vi "CRYAna Harmonic.vi"(0 "Calibration Response Cluster":T1={"Calibration"={"Calibration Step Name"="", "Device"="", "Correction Curve Name"="", "Equalization Curve Name"="", "Sensitivity Curve Name"="", "Corr Folder and File"="", "EQ Folder and File"="", "Sens Folder and File"="", "Corr Step size"=0, "EQ Step size"=0, "Input"=FALSE, "Last Cal Date (sec)"=timestamp(0 s since 1904-01-01), "Cha Name"="", "Corr Curve Found"=FALSE, "EQ Curve Found"=FALSE, "Sens Curve Found"=FALSE, "Signal Type"="", "Calibrated Device"="", "Hz"=0}, "Corr Curve"={"Name"="", "Curve"=[], "X data"=1, "Y data"=1, "Z data"=1, "X axis"=0, "Y axis"=1, "Z axis"=1, "X unit"="Hz", "Y unit"="", "Z unit"="deg.", "X dB ref"=1.0, "Y dB ref"=1.0, "Z dB ref"=1.0, "single val"=FALSE, "protected"=FALSE, "display X"=TRUE, "display Y"=TRUE, "display Z"=TRUE, "Test Info"="", "Step No."=0, "Plot Settings"={"Color"=0, "Interpolation"=0, "Point Style"=0, "Line Style"=0, "Point Color"=0, "Line Width"=0, "Bar Plot Style"=0, "Fill To"=0}, "AutoProtect"=FALSE}, "EQ Curve"={"Name"="", "Curve"=[], "X data"=1, "Y data"=1, "Z data"=1, "X axis"=0, "Y axis"=1, "Z axis"=1, "X unit"="Hz", "Y unit"="", "Z unit"="deg.", "X dB ref"=1.0, "Y dB ref"=1.0, "Z dB ref"=1.0, "single val"=FALSE, "protected"=FALSE, "display X"=TRUE, "display Y"=TRUE, "display Z"=TRUE, "Test Info"="", "Step No."=0, "Plot Settings"={"Color"=0, "Interpolation"=0, "Point Style"=0, "Line Style"=0, "Point Color"=0, "Line Width"=0, "Bar Plot Style"=0, "Fill To"=0}, "AutoProtect"=FALSE}, "Sens Curve"={"Name"="", "Curve"=[], "X data"=1, "Y data"=1, "Z data"=1, "X axis"=0, "Y axis"=1, "Z axis"=1, "X unit"="Hz", "Y unit"="", "Z unit"="deg.", "X dB ref"=1.0, "Y dB ref"=1.0, "Z dB ref"=1.0, "single val"=FALSE, "protected"=FALSE, "display X"=TRUE, "display Y"=TRUE, "display Z"=TRUE, "Test Info"="", "Step No."=0, "Plot Settings"={"Color"=0, "Interpolation"=0, "Point Style"=0, "Line Style"=0, "Point Color"=0, "Line Width"=0, "Bar Plot Style"=0, "Fill To"=0}, "AutoProtect"=FALSE}} {"Sens Curve"."Z data" items=["dB", "Lin"]; "Sens Curve"."X data" items=["dB", "Lin"]; "Sens Curve"."Y data" items=["dB", "Lin"]; "Sens Curve"."Z dB ref" format="%.1f"; "Sens Curve"."Z axis" items=["Log", "Lin"]; "Sens Curve"."X dB ref" format="%.1f"; "Sens Curve"."X axis" items=["Log", "Lin"]; "Sens Curve"."Y axis" items=["Log", "Lin"]; "Sens Curve"."Y dB ref" format="%.1f"; "Sens Curve"."Curve"."z" format="%.2f"; "Sens Curve"."Curve"."y" format="%.2f"; "Sens Curve"."Curve"."x" format="%.2f"; "EQ Curve"."Z data" items=["dB", "Lin"]; "EQ Curve"."X data" items=["dB", "Lin"]; "EQ Curve"."Y data" items=["dB", "Lin"]; "EQ Curve"."Z dB ref" format="%.1f"; "EQ Curve"."Z axis" items=["Log", "Lin"]; "EQ Curve"."X dB ref" format="%.1f"; "EQ Curve"."X axis" items=["Log", "Lin"]; "EQ Curve"."Y axis" items=["Log", "Lin"]; "EQ Curve"."Y dB ref" format="%.1f"; "EQ Curve"."Curve"."z" format="%.2f"; "EQ Curve"."Curve"."y" format="%.2f"; "EQ Curve"."Curve"."x" format="%.2f"; "Corr Curve"."Z data" items=["dB", "Lin"]; "Corr Curve"."X data" items=["dB", "Lin"]; "Corr Curve"."Y data" items=["dB", "Lin"]; "Corr Curve"."Z dB ref" format="%.1f"; "Corr Curve"."Z axis" items=["Log", "Lin"]; "Corr Curve"."X dB ref" format="%.1f"; "Corr Curve"."X axis" items=["Log", "Lin"]; "Corr Curve"."Y axis" items=["Log", "Lin"]; "Corr Curve"."Y dB ref" format="%.1f"; "Corr Curve"."Curve"."z" format="%.2f"; "Corr Curve"."Curve"."y" format="%.2f"; "Corr Curve"."Curve"."x" format="%.2f"; "Calibration"."EQ Step size" items=["R10", "R20", "R40", "R80", "User"]; "Calibration"."Corr Step size" items=["R10", "R20", "R40", "R80", "User"]}, 4 "Distortion Infor":T7, 5 "Calibration Stimulus Cluster":T1={"Calibration"={"Calibration Step Name"="", "Device"="", "Correction Curve Name"="", "Equalization Curve Name"="", "Sensitivity Curve Name"="", "Corr Folder and File"="", "EQ Folder and File"="", "Sens Folder and File"="", "Corr Step size"=0, "EQ Step size"=0, "Input"=FALSE, "Last Cal Date (sec)"=timestamp(0 s since 1904-01-01), "Cha Name"="", "Corr Curve Found"=FALSE, "EQ Curve Found"=FALSE, "Sens Curve Found"=FALSE, "Signal Type"="", "Calibrated Device"="", "Hz"=0}, "Corr Curve"={"Name"="", "Curve"=[], "X data"=1, "Y data"=1, "Z data"=1, "X axis"=0, "Y axis"=1, "Z axis"=1, "X unit"="Hz", "Y unit"="", "Z unit"="deg.", "X dB ref"=1.0, "Y dB ref"=1.0, "Z dB ref"=1.0, "single val"=FALSE, "protected"=FALSE, "display X"=TRUE, "display Y"=TRUE, "display Z"=TRUE, "Test Info"="", "Step No."=0, "Plot Settings"={"Color"=0, "Interpolation"=0, "Point Style"=0, "Line Style"=0, "Point Color"=0, "Line Width"=0, "Bar Plot Style"=0, "Fill To"=0}, "AutoProtect"=FALSE}, "EQ Curve"={"Name"="", "Curve"=[], "X data"=1, "Y data"=1, "Z data"=1, "X axis"=0, "Y axis"=1, "Z axis"=1, "X unit"="Hz", "Y unit"="", "Z unit"="deg.", "X dB ref"=1.0, "Y dB ref"=1.0, "Z dB ref"=1.0, "single val"=FALSE, "protected"=FALSE, "display X"=TRUE, "display Y"=TRUE, "display Z"=TRUE, "Test Info"="", "Step No."=0, "Plot Settings"={"Color"=0, "Interpolation"=0, "Point Style"=0, "Line Style"=0, "Point Color"=0, "Line Width"=0, "Bar Plot Style"=0, "Fill To"=0}, "AutoProtect"=FALSE}, "Sens Curve"={"Name"="", "Curve"=[], "X data"=1, "Y data"=1, "Z data"=1, "X axis"=0, "Y axis"=1, "Z axis"=1, "X unit"="Hz", "Y unit"="", "Z unit"="deg.", "X dB ref"=1.0, "Y dB ref"=1.0, "Z dB ref"=1.0, "single val"=FALSE, "protected"=FALSE, "display X"=TRUE, "display Y"=TRUE, "display Z"=TRUE, "Test Info"="", "Step No."=0, "Plot Settings"={"Color"=0, "Interpolation"=0, "Point Style"=0, "Line Style"=0, "Point Color"=0, "Line Width"=0, "Bar Plot Style"=0, "Fill To"=0}, "AutoProtect"=FALSE}} {"Sens Curve"."Z data" items=["dB", "Lin"]; "Sens Curve"."X data" items=["dB", "Lin"]; "Sens Curve"."Y data" items=["dB", "Lin"]; "Sens Curve"."Z dB ref" format="%.1f"; "Sens Curve"."Z axis" items=["Log", "Lin"]; "Sens Curve"."X dB ref" format="%.1f"; "Sens Curve"."X axis" items=["Log", "Lin"]; "Sens Curve"."Y axis" items=["Log", "Lin"]; "Sens Curve"."Y dB ref" format="%.1f"; "Sens Curve"."Curve"."z" format="%.2f"; "Sens Curve"."Curve"."y" format="%.2f"; "Sens Curve"."Curve"."x" format="%.2f"; "EQ Curve"."Z data" items=["dB", "Lin"]; "EQ Curve"."X data" items=["dB", "Lin"]; "EQ Curve"."Y data" items=["dB", "Lin"]; "EQ Curve"."Z dB ref" format="%.1f"; "EQ Curve"."Z axis" items=["Log", "Lin"]; "EQ Curve"."X dB ref" format="%.1f"; "EQ Curve"."X axis" items=["Log", "Lin"]; "EQ Curve"."Y axis" items=["Log", "Lin"]; "EQ Curve"."Y dB ref" format="%.1f"; "EQ Curve"."Curve"."z" format="%.2f"; "EQ Curve"."Curve"."y" format="%.2f"; "EQ Curve"."Curve"."x" format="%.2f"; "Corr Curve"."Z data" items=["dB", "Lin"]; "Corr Curve"."X data" items=["dB", "Lin"]; "Corr Curve"."Y data" items=["dB", "Lin"]; "Corr Curve"."Z dB ref" format="%.1f"; "Corr Curve"."Z axis" items=["Log", "Lin"]; "Corr Curve"."X dB ref" format="%.1f"; "Corr Curve"."X axis" items=["Log", "Lin"]; "Corr Curve"."Y axis" items=["Log", "Lin"]; "Corr Curve"."Y dB ref" format="%.1f"; "Corr Curve"."Curve"."z" format="%.2f"; "Corr Curve"."Curve"."y" format="%.2f"; "Corr Curve"."Curve"."x" format="%.2f"; "Calibration"."EQ Step size" items=["R10", "R20", "R40", "R80", "User"]; "Calibration"."Corr Step size" items=["R10", "R20", "R40", "R80", "User"]}, 6 "Stimulus Infor":T4, 8 "Time Infor":cluster{"window":u16, "discard cycles":dbl}={"window"=0, "discard cycles"=3.0} {"discard cycles" min=1.0}, 9 "Wave Infor":T6 {"Sens In" format="%.2f"; "Response(Abs/Rel)" items=["Absolute", "Relative"]}, 10 "Response":dbl[](array[numeric]), 11 "Algorithm":u16) -> (1 "Freq resp curves clipped":cluster{cluster{"x":dbl, "y":dbl, "z":dbl}[]}[](array[cluster]), 2 "Harmonic Track Out":T5(array[cluster]))   [LabVIEW 2013]
uses:
  Typedef Control/CRYCalibration 2DCluster.ctl
  Typedef Control/CRYCalibration Cluster.ctl
  Typedef Control/CRYData Cluster.ctl
  <vilib>/Analysis/2dsp.llb/Real FFT.vi
  <vilib>/Analysis/2dsp.llb/Zero Padder (DBL).vi
  <vilib>/Analysis/NI_AALPro.lvlib
panel:
  # "* measurement confidence\n0. Standard Error\n1. Confidence Limits\n2. Total Noise\n\n*Harmonics\n3. Harmonics @meas.Frq\n4. Total Distortion\n5. THD [%]\n6. THD Normalized [%]\n7. THD + Noise [%]\n8. Rub & Buzz [%]\n9. Rub & Buzz Norm'd [%]\n\nIM\n10. Total IM\n11. Total IM [%]\n12. Total IM + Noise [%]\n\nDiff\n13. Total Diff\n14. Total DFD [%]\n15. Total DFD + Noise [%]"
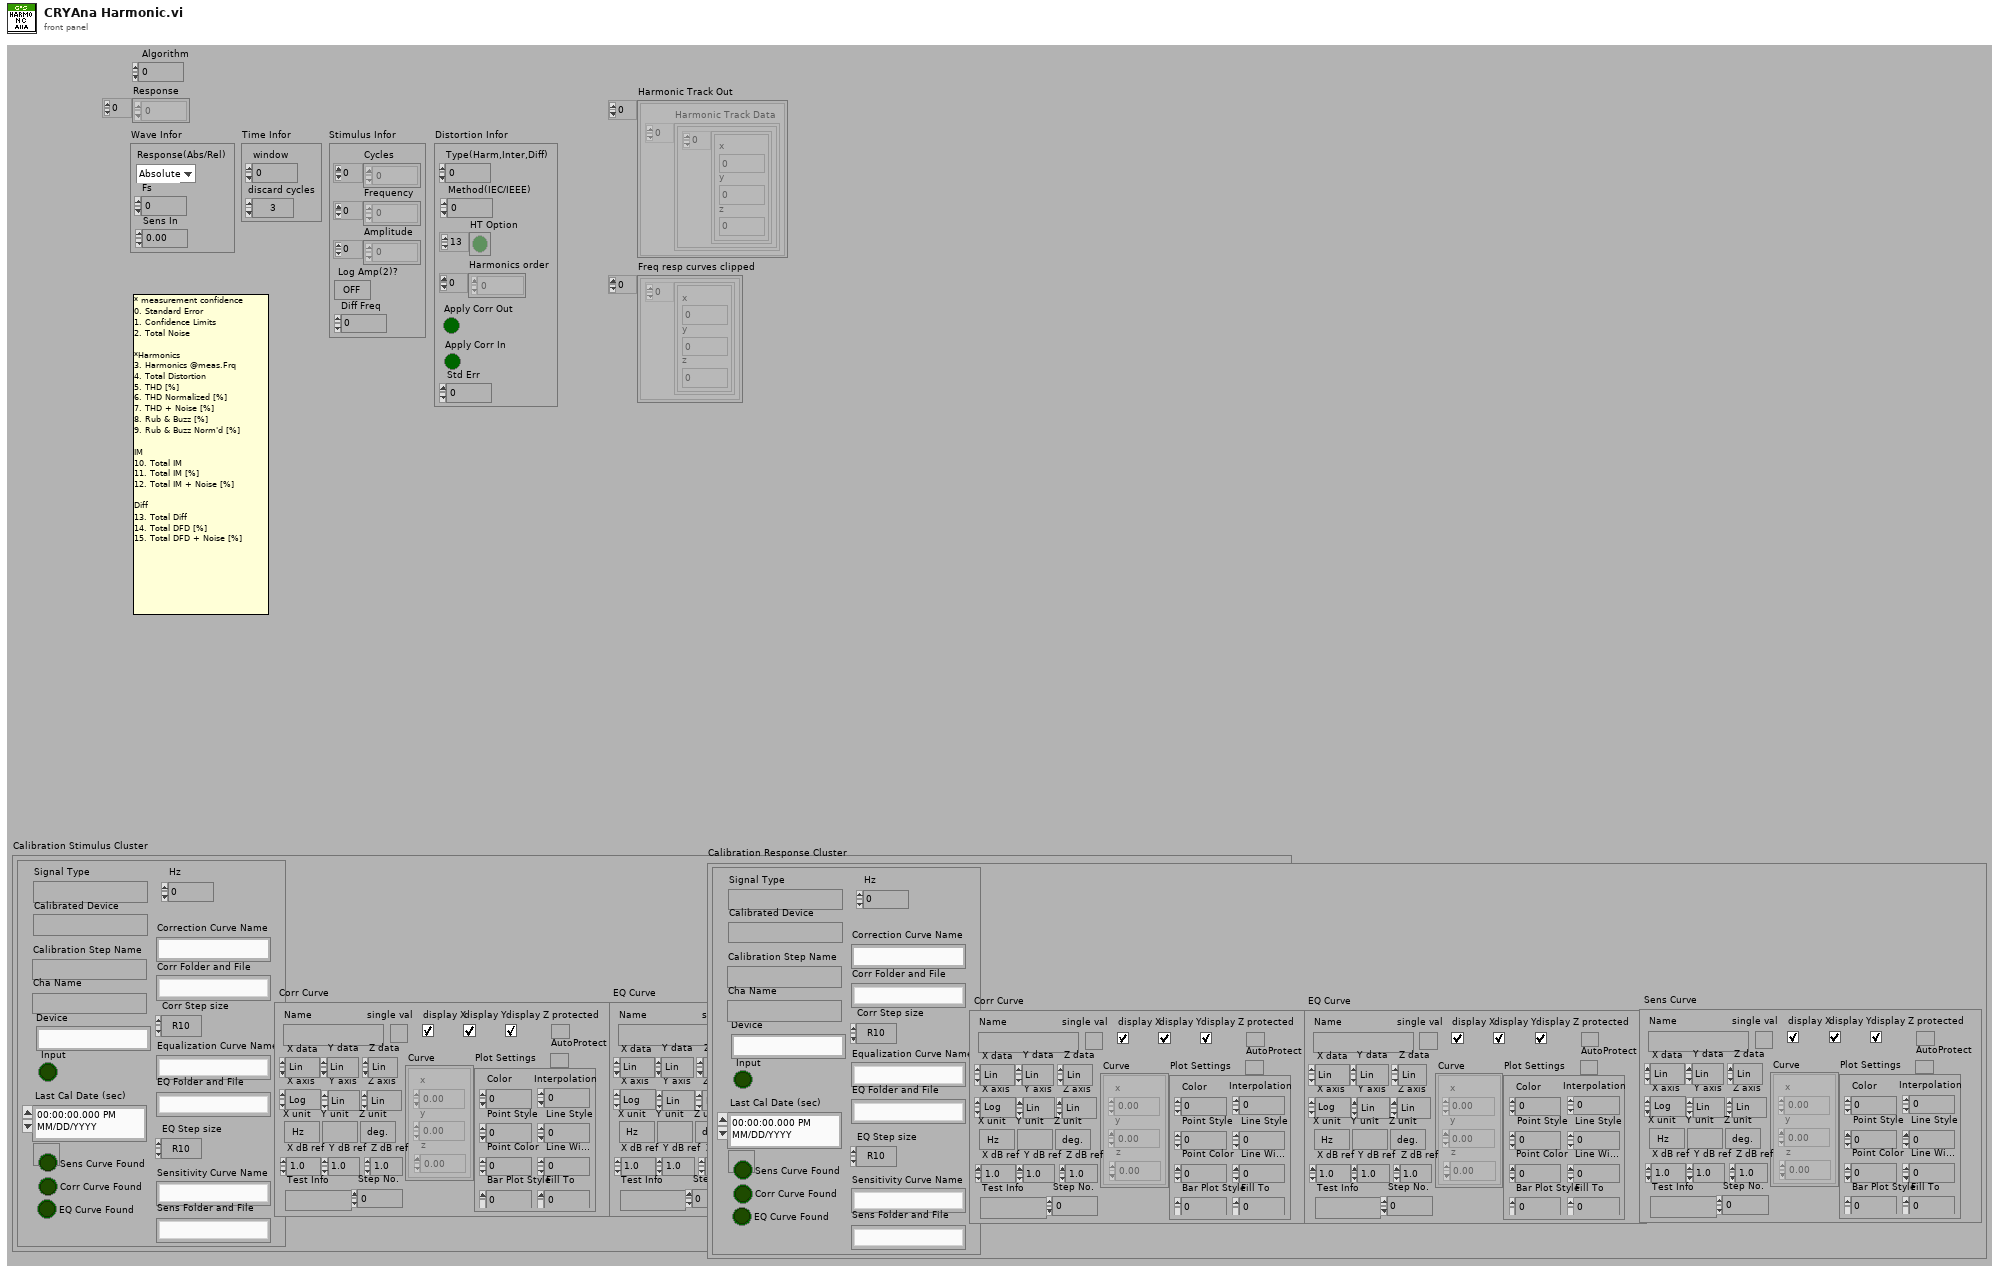
[diagram p1: front panel]
types:
  T1 = typedef "CRYCalibration 2DCluster.ctl" = cluster{"Calibration":T2, "Corr Curve":T3, "EQ Curve":T3, "Sens Curve":T3}
  T2 = typedef "CRYCalibration Cluster.ctl" = cluster{"Calibration Step Name":string, "Device":string, "Correction Curve Name":string, "Equalization Curve Name":string, "Sensitivity Curve Name":string, "Corr Folder and File":string, "EQ Folder and File":string, "Sens Folder and File":string, "Corr Step size":u16, "EQ Step size":u16, "Input":bool, "Last Cal Date (sec)":timestamp, "Cha Name":string, "Corr Curve Found":bool, "EQ Curve Found":bool, "Sens Curve Found":bool, "Signal Type":string, "Calibrated Device":string, "Hz":u32}
  T3 = typedef "CRYData Cluster.ctl" = cluster{"Name":string, "Curve":cluster{"x":dbl, "y":dbl, "z":dbl}[], "X data":u16, "Y data":u16, "Z data":u16, "X axis":u16, "Y axis":u16, "Z axis":u16, "X unit":string, "Y unit":string, "Z unit":string, "X dB ref":dbl, "Y dB ref":dbl, "Z dB ref":dbl, "single val":bool, "protected":bool, "display X":bool, "display Y":bool, "display Z":bool, "Test Info":string, "Step No.":i32, "Plot Settings":cluster{"Color":u32, "Interpolation":u8, "Point Style":u8, "Line Style":u8, "Point Color":u32, "Line Width":u8, "Bar Plot Style":u8, "Fill To":i16}, "AutoProtect":bool}
  T4 = cluster{"Cycles":dbl[], "Frequency":dbl[], "Amplitude":dbl[], " Log Amp(2)?":bool, "Diff Freq":dbl}
  T5 = cluster{"Harmonic Track Data":cluster{cluster{"x":dbl, "y":dbl, "z":dbl}[]}[]}[]
  T6 = cluster{"Response(Abs/Rel)":u16, "Fs":dbl, "Sens In":dbl}
  T7 = cluster{"Type(Harm,Inter,Diff)":u16, "Method(IEC/IEEE)":u16, "HT Option":bool[], "Harmonics order":dbl[], "Apply Corr Out":bool, "Apply Corr In":bool, "Std Err":dbl}
  T8 = cluster{"Fi":dbl, "element":dbl, "element":dbl}[]
  T9 = cluster{cluster{"Fi":dbl, "element":dbl, "element":dbl}[]}
  T10 = cluster{"Harmonic Track Data":cluster{cluster{"x":dbl, "y":dbl, "z":dbl}[]}[]}
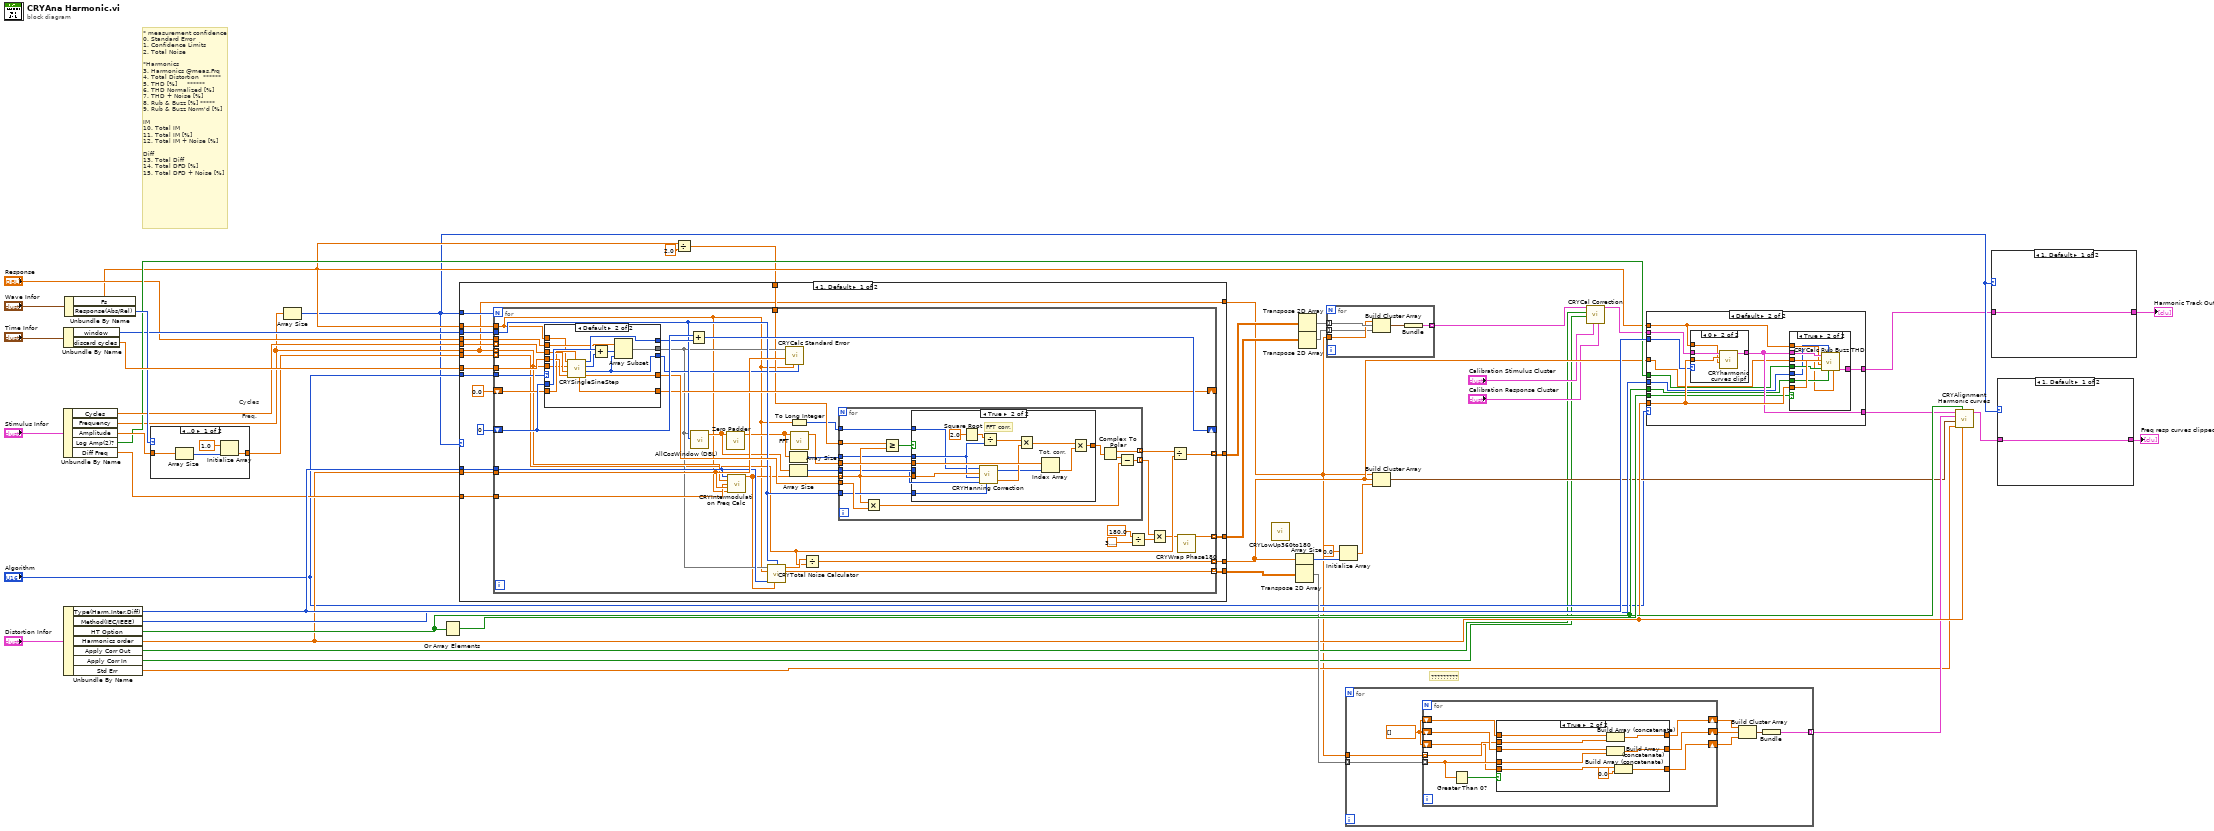
[diagram p0: block diagram]
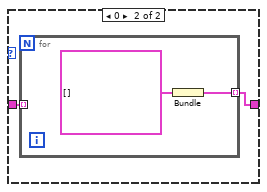
[diagram p2: hidden frame]
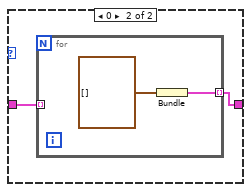
[diagram p3: hidden frame]
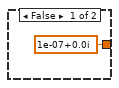
[diagram p4: hidden frame]
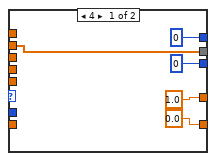
[diagram p5: hidden frame]
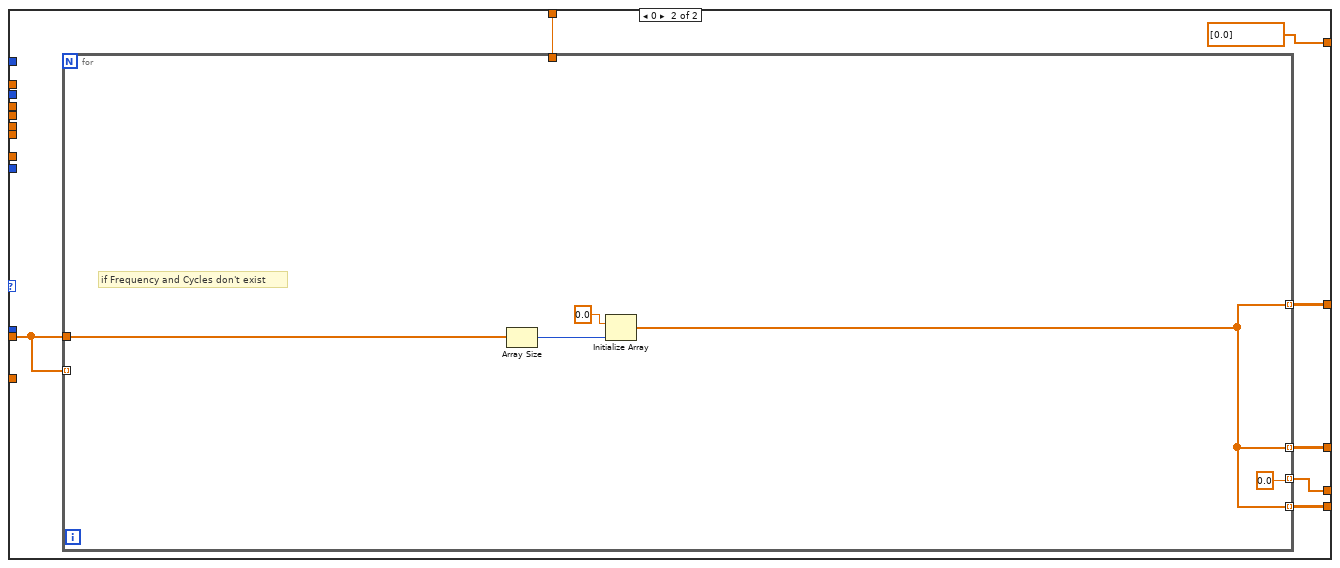
[diagram p6: hidden frame]
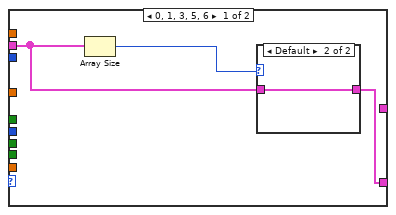
[diagram p9: hidden frame]
diagram:
  # "* measurement confidence\n0. Standard Error\n1. Confidence Limits\n2. Total Noise\n\n*Harmonics\n3. Harmonics @meas.Frq\n4. Total Distortion  ******\n5. THD [%]     ******\n6. THD Normalized [%]\n7. THD + Noise [%]\n8. Rub & Buzz [%] *****\n9. Rub & Buzz Norm'd [%]\n\nIM\n10. Total IM\n11. Total IM [%]\n12. Total IM + Noise [%]\n\nDiff\n13. Total Diff\n14. Total DFD [%]\n15. Total DFD + Noise [%]"
  # "?????????"
  # "Cycles"
  # "Freq."
  n1 = Unbundle By Name("Stimulus Infor") -> ("Cycles"=w39:dbl[], "Frequency"=w26:dbl[], "Amplitude"=w38:dbl[], "Log Amp(2)?"=w37:bool, "Diff Freq"=w36:dbl)
  n2 = Unbundle By Name("Time Infor") -> ("window"=w34:u16, "discard cycles"=w46:dbl)
  n3 = Unbundle By Name("Distortion Infor") -> ("Type(Harm,Inter,Diff)"=w44:u16, "Method(IEC/IEEE)"=w43:u16, "HT Option"=w29:bool[], "Harmonics order"=w28:dbl[], "Apply Corr Out"=w13:bool, "Apply Corr In"=w12:bool, "Std Err"=w10:dbl)
  n4 = Unbundle By Name("Wave Infor") -> ("Fs"=w8:dbl, "Response(Abs/Rel)"=w41:u16)
  n5 = case shown="..0" w41 {
    tunnel: [w50 w54] -> w35
    tunnel: w38 -> [w53 w54]
    frame ..0 {
      n6 = Array Size(array=w53) -> (size(s)=w52:i32)
      n7 = Initialize Array(1.0 ("Level left"), w52) -> (w50:dbl[])
    }
    frame 1.. {
    }
  }
  n8 = Array Size(array=w26) -> (size(s)=w3:i32)
  n9 = Or Array Elements(Boolean array=w29) -> (logical OR=w48:bool)
  n10 = Divide(x=w8, y=2.0) -> (x/y=w7:dbl)
  n11 = case shown="1, Default" w3 {
    tunnel: w3 -> [w72 _]
    tunnel: [w71 w166] -> w49
    tunnel: w46 -> [w69 _]
    tunnel: w44 -> [w68 _]
    tunnel: w39 -> [w67 _]
    tunnel: w36 -> [w66 _]
    tunnel: w35 -> [w65 _]
    tunnel: w34 -> [w64 _]
    tunnel: [w63 w165] -> w33
    tunnel: [w62 w164] -> w32
    tunnel: "Response" -> [w61 _]
    tunnel: w28 -> [w60 w161]
    tunnel: w26 -> [w55 _]
    tunnel: [w59 w163] -> w23
    tunnel: "Algorithm" -> [w58 _]
    tunnel: w8 -> [w57 _]
    tunnel: w7 -> [w56 w162]
    tunnel: [w55 dbl[] [0.0] ("Frequency")] -> w6
    frame 1, Default {
      n12 = for {
        N: w72 -> [_]
        tunnel: w57 -> [w78]
        shift-right: [w107] -> _
        shift-left: 0 -> [w106]
        tunnel: w61 -> [w94]
        tunnel: w67 -> [w104] mode=indexing
        tunnel: w58 -> [w90]
        tunnel: w55 -> [w95] mode=indexing
        tunnel: [w108] -> w63 mode=indexing
        tunnel: [w74] -> w71 mode=indexing
        tunnel: w60 -> [w98]
        tunnel: w65 -> [w87] mode=indexing
        tunnel: w69 -> [w103]
        shift-right: [w99] -> _
        shift-left: 0.0 -> [w102]
        tunnel: w68 -> [w97]
        tunnel: [w86] -> w59 mode=indexing
        tunnel: w66 -> [w96]
        tunnel: w64 -> [w92]
        tunnel: [w93] -> w62 mode=indexing
        tunnel: w56 -> [w83]
        n13 = case shown="Default" w90 {
          tunnel: w106 -> [_ w159]
          tunnel: w104 -> [_ w158]
          tunnel: w103 -> [_ w157]
          tunnel: w102 -> [_ w156]
          tunnel: [0 ("TotalSamples") w155] -> w101
          tunnel: [1.0 ("TimeCorrection") w154] -> w100
          tunnel: [0.0 ("StopPhase") w153] -> w99
          tunnel: w95 -> [_ w152]
          tunnel: w94 -> [w141 w151]
          tunnel: w78 -> [_ w150]
          tunnel: [w141 w148] -> w89
          tunnel: [0 ("ExtractSamples") w147] -> w91
          frame 4 {
          }
          frame Default {
            n14 = call "CRYSingleSineStep.vi"("Fs"=w150, "Freq"=w152, "Cycles per freq"=w158, "Cycles discarded"=w157, "StartPhase"=w156) -> ("StopPhase"=w153:dbl, "TotalSamples"=w155:i32, "DiscardSamples"=w146:i32, "ExtractSamples"=w147:i32, "TimeCorrection"=w154:dbl)  [unwired: 1 out]
            n15 = Add(x=w159, y=w146) -> (x+y=w149:i32)
            n16 = Array Subset(array=w151, index=w149, length=w147) -> (w148:dbl[])
          }
        }
        n17 = Add(x=w106, y=w101) -> (x+y=w107:i32)
        n18 = call <vilib>:"AllCosWindow (DBL).vi"("window"=w92, "X"=w89) -> ("Windowed X"=w82:dbl[])  [unwired: 1 in, 3 out]
        n19 = call-poly <vilib>:"Zero Padder.vi"("Input Array"=w82) -> ("Zero Padded Array"=w81:dbl[])  [unwired: 1 in, 9 out]
        n20 = call "CRYIntermodulation Freq Calc.vi"("Type"=w97, "Freq1 In"=w95, "Freq2 In"=w96, "Orders"=w98, "Fs"=w78) -> ("Frequency Array Out"=w85:dbl[])  [unwired: 10 in]
        n21 = call "CRYTotal Noise Calculator.vi"("Input Signal"=w89, "window"=w92, "Fs"=w78, "Type(Harm,Inter,Diff)"=w97, "Freq Array"=w85) -> ("Total Noise"=w88:dbl, "Standard Error"=w93:dbl[])  [unwired: 9 in]
        n22 = call "CRYCalc Standard Error.vi"("N(Samples #)"=w91, "Fs"=w78, "Harmonic Frequency"=w98, "X(t)"=w89) -> ()  [unwired: 8 in]
        n23 = Array Size(array=w81) -> (size(s)=w80:i32)
        n24 = Array Size(array=w82) -> (size(s)=w79:i32)
        n25 = To Long Integer(number=w78) -> (32bit integer=w77:i32)
        n26 = call-poly <vilib>:"FFT.vi"("X"=w81) -> ("FFT {X}"=w84:cdb[])  [unwired: 2 in, 8 out]
        n27 = Divide(x=w88, y=w87) -> (x/y=w86:dbl)
        n28 = for {
          tunnel: w84 -> [w124]
          tunnel: [w114] -> w110 mode=indexing
          tunnel: [w121] -> w109 mode=indexing
          tunnel: w83 -> [w122]
          tunnel: w100 -> [w118]
          tunnel: w77 -> [w117]
          tunnel: w85 -> [w115] mode=indexing
          tunnel: w92 -> [w116]
          tunnel: w80 -> [w113]
          tunnel: w79 -> [w112]
          n29 = Multiply(x=w115, y=w118) -> (x*y=w119:dbl)
          n30 = Greater Or Equal?(x=w122, y=w115) -> (x >= y?=w123:bool)
          n31 = case shown="True" w123 {
            tunnel: w124 -> [_ w140]
            tunnel: [cdb 1e-07+0.0i w130] -> w125
            tunnel: w115 -> [_ w131]
            tunnel: w117 -> [_ w127]
            tunnel: w116 -> [_ w132]
            tunnel: w113 -> [_ w129]
            tunnel: w112 -> [_ w128]
            frame False {
            }
            frame True {
              # "Tot. corr."
              # "FFT corr."
              n32 = Square Root(x=2.0) -> (sqrt(x)=w135:dbl)
              n33 = call "CRYHanning Correction.vi"("window"=w132, "N sine"=w128, "N FFT"=w129, "frequency"=w131, "Fs"=w127) -> ("Complex correction factor"=w137:cdb, "Index sine"=w133:i32)  [unwired: 1 out]
              n34 = Divide(x=w135, y=w129) -> (x/y=w136:dbl)
              n35 = Multiply(x=w136, y=w137) -> (x*y=w138:cdb)
              n36 = Index Array(array=w140, index=w133) -> (element=w139:cdb)
              n37 = Multiply(x=w138, y=w139) -> (x*y=w130:cdb)
            }
          }
          n38 = Complex To Polar(r * e^(i*theta)=w125) -> (r=w114:dbl, theta=w120:dbl)
          n39 = Subtract(x=w120, y=w119) -> (x-y=w121:dbl)
        }
        n40 = Divide(x=180.0, y=3.141592653589793) -> (x/y=w105:dbl)
        n41 = Multiply(x=w109, y=w105) -> (x*y=w75:dbl[])
        n42 = Divide(x=w110, y=w87) -> (x/y=w108:dbl[])
        n43 = call "CRYWrap Phase180.vi"("Phase In"=w75) -> ("Phase Out"=w74:dbl[])  [unwired: 10 in]
      }
    }
    frame 0 {
      n44 = for {
        tunnel: [w169] -> w165 mode=indexing
        tunnel: [w169] -> w166 mode=indexing
        tunnel: w161 -> [w167]
        tunnel: [0.0] -> w163 mode=indexing
        tunnel: [w169] -> w164 mode=indexing
        tunnel: w162 -> [_]
        tunnel: w161 -> [_] mode=indexing
        # "if Frequency and Cycles don't exist"
        n45 = Array Size(array=w167) -> (size(s)=w171:i32)
        n46 = Initialize Array(0.0 ("element"), w171) -> (w169:dbl[])
      }
    }
  }
  n47 = call "CRYLowUp360to180.vi"() -> ()  [unwired: 11 in, 1 out]
  n48 = Array Size(array=w23) -> (size(s)=w24:i32)
  n49 = Transpose 2D Array(2D array=w32) -> (transposed array=w31:dbl[][])
  n50 = Transpose 2D Array(2D array=w33) -> (transposed array=w19:dbl[][])
  n51 = Transpose 2D Array(2D array=w49) -> (transposed array=w20:dbl[][])
  n52 = for {
    tunnel: w19 -> [w176] mode=indexing
    tunnel: w20 -> [w172] mode=indexing
    tunnel: w6 -> [w175]
    tunnel: [w173] -> w17 mode=indexing
    n53 = Build Cluster Array(w175, w176, w172) -> (w174:T8)
    n54 = Bundle(w174) -> (w173:T9)  [unwired: 1 in]
  }
  n55 = Initialize Array(0.0 ("element"), w24) -> (w18:dbl[])
  n56 = for {
    tunnel: w6 -> [w184]
    tunnel: w31 -> [w183] mode=indexing
    tunnel: [w182] -> w27 mode=indexing
    w181 = dbl[] []
    n57 = for {
      tunnel: w183 -> [w188] mode=indexing
      tunnel: w184 -> [w189] mode=indexing
      shift-right: [w192] -> w180
      shift-left: w181 -> [w193]
      shift-right: [w190] -> w179
      shift-left: w181 -> [w191]
      shift-right: [w185] -> w177
      shift-left: w181 -> [w186]
      n58 = Greater Than 0?(x=w188) -> (x > 0?=w187:bool)
      n59 = case shown="True" w187 {
        tunnel: w188 -> [_ w205]
        tunnel: w193 -> [w196 w204]
        tunnel: [w196 w203] -> w192
        tunnel: w191 -> [w195 w202]
        tunnel: [w195 w201] -> w190
        tunnel: w189 -> [_ w200]
        tunnel: w186 -> [w194 w199]
        tunnel: [w194 w197] -> w185
        frame False {
        }
        frame True {
          n60 = Build Array (concatenate)(w204, w200) -> (w203:dbl[])
          n61 = Build Array (concatenate)(w202, w205) -> (w201:dbl[])
          n62 = Build Array (concatenate)(w199, 0.0 ("rms value")) -> (w197:dbl[])
        }
      }
    }
    n63 = Build Cluster Array(w180, w179, w177) -> (w178:cluster{"Fi":dbl, "Fi":dbl, "Fi":dbl}[])
    n64 = Bundle(w178) -> (w182:cluster{cluster{"Fi":dbl, "Fi":dbl, "Fi":dbl}[]})  [unwired: 1 in]
  }
  n65 = Build Cluster Array(w6, w23, w18) -> (w25:cluster{"Fi":dbl, dbl, "element":dbl}[])
  n66 = call "CRYCal Correction.vi"("Calibration Response Cluster"="Calibration Response Cluster", "Calibration Stimulus Cluster"="Calibration Stimulus Cluster", "Apply Corr In"=w12, "Apply Corr Out"=w13, "Frequency curve in"=w17) -> ("Frequency curve out"=w16:cluster{cluster{"x":dbl, "y":dbl, "z":dbl}[]}[])  [unwired: 6 in]
  n67 = case shown="Default" "Algorithm" {
    tunnel: w28 -> [_ w220]
    tunnel: [w206 w219] -> w11
    tunnel: w37 -> [_ w218]
    tunnel: w16 -> [w207 w217]
    tunnel: w48 -> [_ w216]
    tunnel: w8 -> [_ w215]
    tunnel: w29 -> [_ w214]
    tunnel: [_ w213] -> w2
    tunnel: w23 -> [_ w212]
    tunnel: w44 -> [_ w211]
    tunnel: w43 -> [_ w210]
    frame 0, 1, 3, 5, 6 {
      n68 = Array Size(array=w207) -> (size(s)=w208:i32)
      n69 = case shown="Default" w208 {
        tunnel: w207 -> [_ w209]
        tunnel: [_ w209] -> w206
        frame 0 {
        }
        frame Default {
        }
      }
    }
    frame Default {
      n70 = case shown="0" w211 {
        tunnel: w220 -> [_ w225]
        tunnel: [w221 w224] -> w219
        tunnel: w217 -> [w221 w223]
        tunnel: w215 -> [_ w222]
        frame Default {
        }
        frame 0 {
          n71 = call "CRYharmonic curves clipf.vi"("Fs"=w222, "Harmonics"=w225, "Freq resp curves"=w223) -> ("Freq resp curves clipped"=w224:cluster{cluster{"x":dbl, "y":dbl, "z":dbl}[]}[])  [unwired: 8 out]
        }
      }
      n72 = case shown="True" w216 {
        tunnel: w219 -> [_ w233]
        tunnel: w220 -> [_ w232]
        tunnel: w215 -> [_ w231]
        tunnel: w218 -> [_ w230]
        tunnel: w214 -> [_ w229]
        tunnel: [_ w228] -> w213
        tunnel: w212 -> [_ w227]
        tunnel: w210 -> [_ w226]
        frame False {
        }
        frame True {
          n73 = call "CRYCalc Rub Buzz THD.vi"("Total Noise"=w227, "HT Option"=w229, "Method"=w226, "Amplitude sweep (F)"=w230, "Fs"=w231, "Harmonics"=w232, "Freq resp curves"=w233) -> ("Harmonic Track Out"=w228:T5)  [unwired: 4 out]
        }
      }
    }
  }
  n74 = call "CRYAlignment Harmonic curves.vi"("Harmonics order"=w28, "HT Option"=w29, "Std Error"=w10, "Total Noise"=w25, "Standard Error"=w27, "Harmonic Curves"=w11) -> ("Freq Curves Out"=w5:cluster{cluster{"x":dbl, "y":dbl, "z":dbl}[]}[])  [unwired: 5 in]
  n75 = case shown="1, Default" w3 {
    tunnel: w2 -> [w234 w236]
    tunnel: [w234 w235] -> w1
    frame 1, Default {
    }
    frame 0 {
      n76 = for {
        tunnel: w236 -> [_] mode=indexing
        tunnel: [w238] -> w235 mode=indexing
        n77 = Bundle("Harmonic Track Data"=cluster{cluster{"x":dbl, "y":dbl, "z":dbl}[]}[] []) -> (w238:T10)  [unwired: 1 in]
      }
    }
  }
  "Harmonic Track Out" <- w1
  n78 = case shown="1, Default" w3 {
    tunnel: w5 -> [w239 w241]
    tunnel: [w239 w240] -> w4
    frame 1, Default {
    }
    frame 0 {
      n79 = for {
        tunnel: w241 -> [_] mode=indexing
        tunnel: [w242] -> w240 mode=indexing
        n80 = Bundle(cluster{"x":dbl, "y":dbl, "z":dbl}[] []) -> (w242:cluster{cluster{"x":dbl, "y":dbl, "z":dbl}[]})  [unwired: 1 in]
      }
    }
  }
  "Freq resp curves clipped" <- w4
